vi "ToGraphVizString.vi"(9 "AST in":refnum<class "VI_AST.lvclass">) -> (3 "AST out":refnum<class "VI_AST.lvclass">, 4 "GraphViz string":string)   [LabVIEW 2014, in "Raspberry Pi Compatible Compiler for LabVIEW.lvlib" / "VI_AST.lvclass"]
uses:
  VI_AST.lvclass
  VI_AST.lvclass/VI_AST.ctl
  DAG/DAG/DAG.lvclass/DAG.ctl
  DAG/DAG/DAG.lvclass
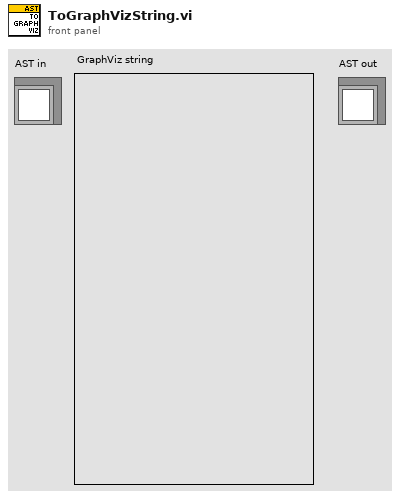
[diagram p1: front panel]
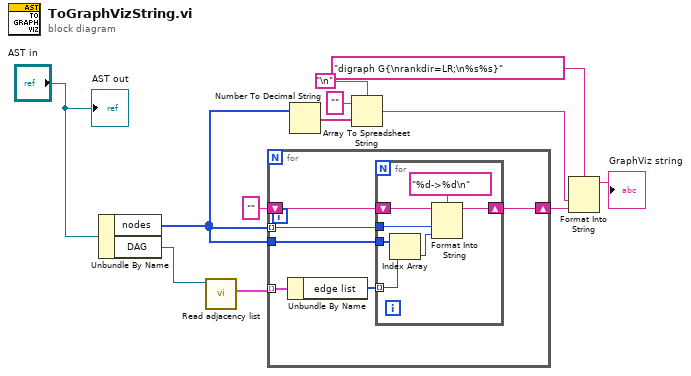
[diagram p0: block diagram]
diagram:
  n1 = Unbundle By Name("AST in") -> ("nodes"=w6:i32[], "DAG"=w8:refnum<class "DAG.lvclass">)
  n2 = call "Read adjacency list.vi"("DAG in"=w8) -> ("adjacency list"=w7:cluster{"edge list":i32[]}[])  [unwired: 9 in, 1 out]
  n3 = for {
    tunnel: w7 -> [w18] mode=indexing
    shift-right: [w16] -> w10
    shift-left: "" -> [w15]
    tunnel: w6 -> [w14] mode=indexing
    tunnel: w6 -> [w13]
    n4 = Unbundle By Name(w18) -> ("edge list"=w17:i32[])
    n5 = for {
      tunnel: w17 -> [w20] mode=indexing
      tunnel: w14 -> [w22]
      shift-right: [w24] -> w16
      shift-left: w15 -> [w23]
      tunnel: w13 -> [w21]
      n6 = Index Array(array=w21, index=w20) -> (element=w19:i32)
      n7 = Format Into String(format string="%d->%d\n", initial string=w23, w22, w19) -> (resulting string=w24:string)  [unwired: 1 in, 1 out]
    }
  }
  n8 = Number To Decimal String(number=w6) -> (decimal integer string=w4:string[])  [unwired: 1 in]
  n9 = Array To Spreadsheet String(delimiter (Tab)="\n", array=w4, 3:"" ("format string")) -> (spreadsheet string=w1:string)
  n10 = Format Into String(format string="digraph G{\nrankdir=LR;\n%s%s}", w1, w10) -> (resulting string=→"GraphViz string":string)  [unwired: 2 in, 1 out]
  "AST out" <- "AST in"
